vi "Create Parameters.vi"(8 "error in (no error)":errorcluster, 10 "Parameters":cluster{"Name":string, "Value":string}[](array[cluster]), 11 "XML Handler in":refnum<class "XML Handler.lvclass">) -> (0 "error out":errorcluster, 3 "XML Handler out":refnum<class "XML Handler.lvclass">)   [LabVIEW 2020, in "XML Handler.lvclass"]
uses:
  XML Handler.lvclass
  XML Handler.lvclass/XML Handler.ctl
  <vilib>/xml/Close Reference(Node).vi
  <resource>/objmgr/DOMUserDefRef.rc
  <vilib>/xml/NI_XML.lvlib
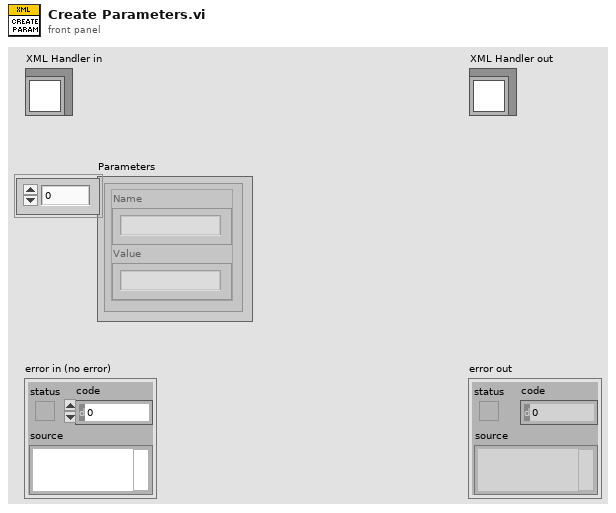
[diagram p1: front panel]
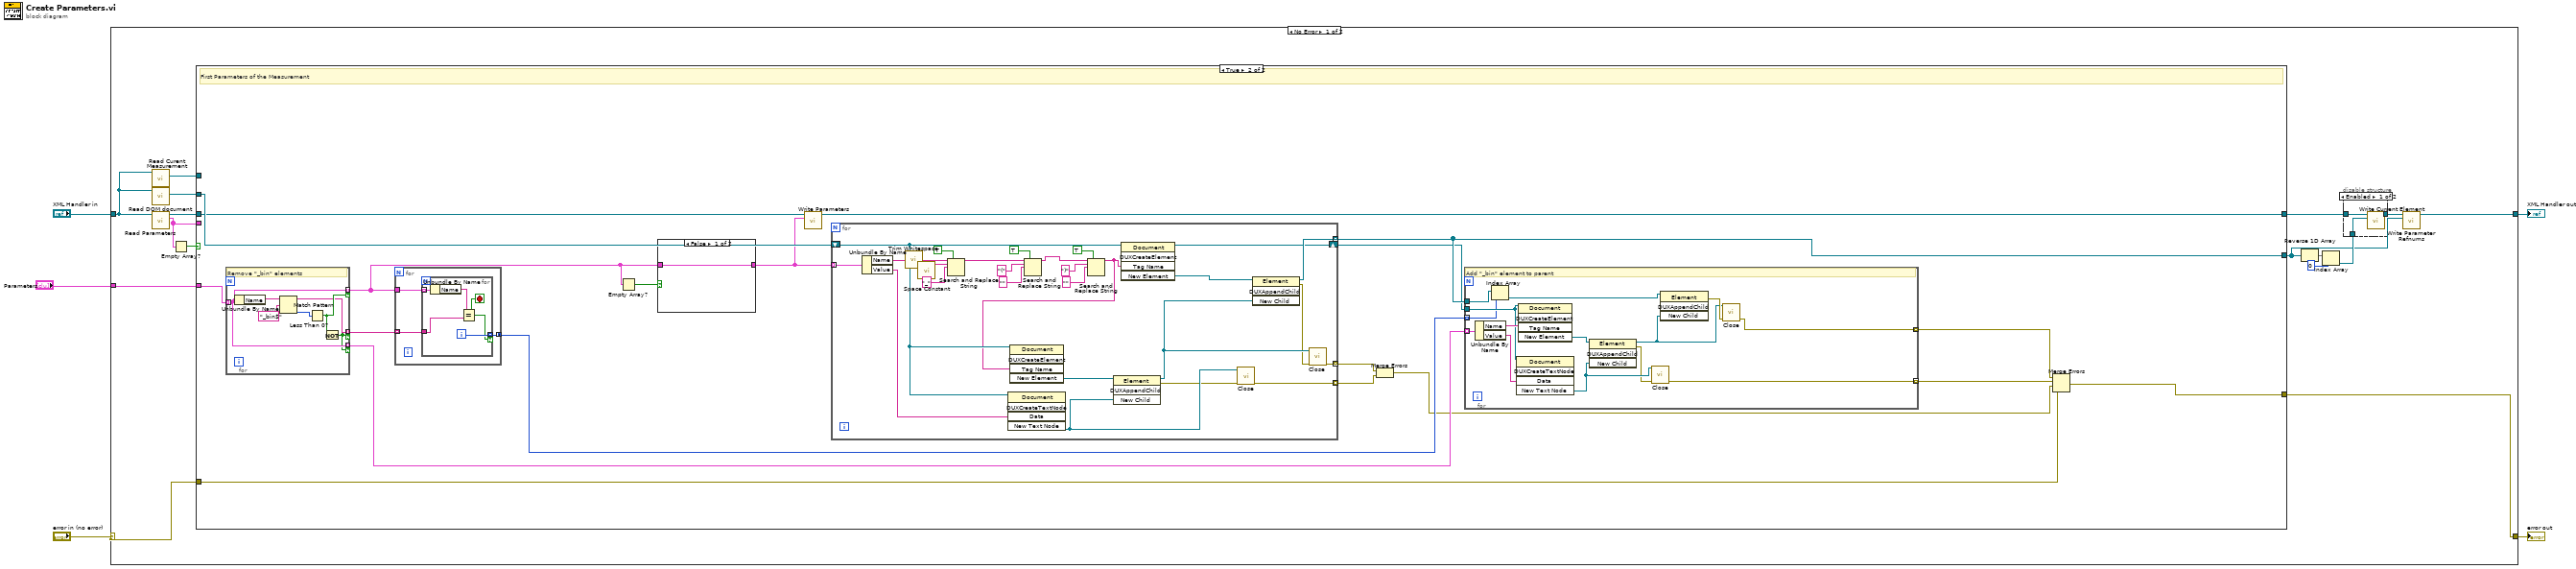
[diagram p0: block diagram]
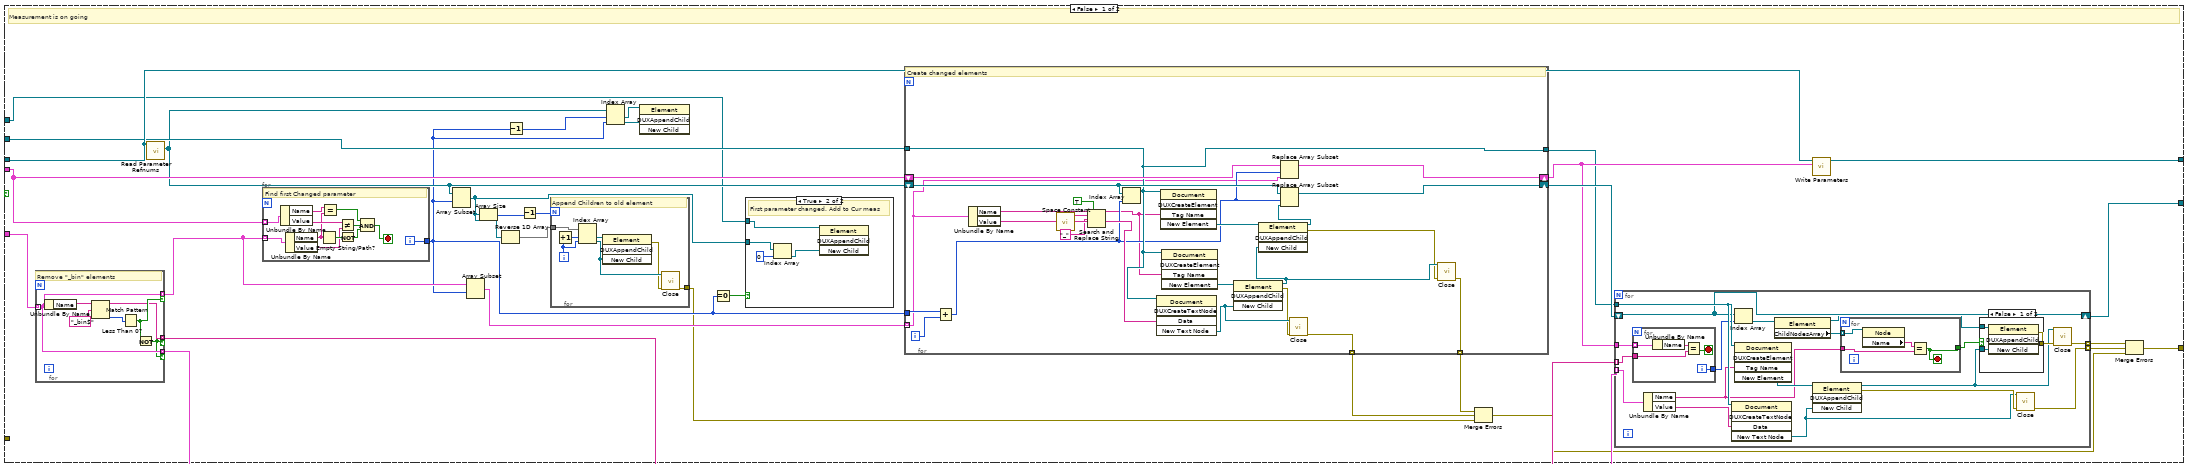
[diagram p3: hidden frame]
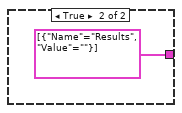
[diagram p6: hidden frame]
diagram:
  n1 = case shown="No Error" "error in (no error)" {
    selector: "error in (no error)" -> [w7 w220]
    tunnel: [w6 w220] -> w4
    tunnel: [w11 w219] -> w2
    tunnel: "XML Handler in" -> [w21 w219]
    tunnel: "Parameters" -> [w20 _]
    frame No Error {
      n2 = call "Read Curent Measurement.vi"("XML Handler in"=w21) -> ("Curent Measurement"=w13:refnum<k20>)  [unwired: 9 in, 1 out]
      n3 = call "Read DOM document.vi"("XML Handler in"=w21) -> ("DOM document"=w15:refnum<k20>)  [unwired: 9 in, 1 out]
      n4 = call "Read Parameters.vi"("XML Handler in"=w21) -> ("Parameters"=w14:cluster{"Name":string, "Value":string}[], "XML Handler out"=w16:refnum<class "XML Handler.lvclass">)  [unwired: 9 in]
      n5 = Empty Array?(array=w14) -> (empty?=w17:bool)
      n6 = case shown="True" w17 {
        tunnel: w16 -> [w55 w159]
        tunnel: w20 -> [w54 w157]
        tunnel: w15 -> [w52 w160]
        tunnel: [w50 w153] -> w10
        tunnel: [w56 w158] -> w18
        tunnel: w14 -> [w53 _]
        tunnel: w13 -> [w34 _]
        tunnel: w7 -> [_ w143]
        tunnel: [w27 w142] -> w6
        frame False {
          # "Measurement is on going"
          n7 = for {
            tunnel: w54 -> [w101] mode=indexing
            tunnel: [w101] -> w45 mode=indexing if=w102
            tunnel: [w101] -> w47 mode=indexing if=w99
            tunnel: [w100] -> w48 mode=indexing if=w99
            # "Remove \"_bin\" elements"
            n8 = Unbundle By Name(w101) -> ("Name"=w105:string)
            n9 = Match Pattern(string=w105, regular expression="_bin$") -> (before substring=w100:string, offset past match=w103:i32)  [unwired: 1 in, 2 out]
            n10 = Less Than 0?(x=w103) -> (x < 0?=w102:bool)
            n11 = Not(x=w102) -> (.not. x?=w99:bool)
          }
          n12 = call "Read Parameter Refnums.vi"("XML Handler in"=w55) -> ("Parameter Refnums"=w41:refnum<k20>[])  [unwired: 9 in, 1 out]
          n13 = for {
            tunnel: w53 -> [w137] mode=indexing
            tunnel: w45 -> [w132] mode=indexing
            tunnel: [w138] -> w37
            i -> [w138]
            stop <- w130 stop-if-true
            # "Find first Changed parameter"
            n14 = Unbundle By Name(w137) -> ("Name"=w134:string, "Value"=w135:string)
            n15 = Unbundle By Name(w132) -> ("Name"=w131:string, "Value"=w136:string)
            n16 = Empty String/Path?(string/path=w131) -> (empty?=w141:bool)
            n17 = Equal?(x=w134, y=w131) -> (x = y?=w133:bool)
            n18 = Not Equal?(x=w135, y=w136) -> (x != y?=w139:bool)
            n19 = Not(x=w141) -> (.not. x?=w140:bool)
            n20 = Compound Arithmetic op=AND(w133, w139, w140) -> (w130:bool)
          }
          n21 = Array Subset(array=w41, index=w37) -> (w35:refnum<k20>[])  [unwired: 1 in]
          n22 = Array Subset(array=w45, index=w37) -> (w42:cluster{"Name":string, "Value":string}[])  [unwired: 1 in]
          n23 = Array Size(array=w35) -> (size(s)=w44:i32)
          n24 = Reverse 1D Array(array=w35) -> (reversed array=w43:refnum<k20>[])
          n25 = Decrement(x=w37) -> (x-1=w40:i32)
          n26 = Decrement(x=w44) -> (x-1=w26:i32)
          n27 = for {
            N: w26 -> [_]
            tunnel: w43 -> [w67]
            tunnel: [w61] -> w31
            i -> [w65]
            # "Append Children to old element"
            n28 = Increment(x=w65) -> (x+1=w66:i32)
            n29 = Index Array(array=w67, index #1=w66, index #2=w65) -> (element #1=w64:refnum<k20>, element #2=w63:refnum<k20>)
            n30 = invoke class="Element" method="DUXAppendChild"(reference=w64, "New Child"=w63) -> (error out=w62:errorcluster)  [unwired: 2 in, 3 out]
            n31 = call-poly <vilib>:"Close.vi"("error in (no error)"=w62, "node"=w63) -> ("error out"=w61:errorcluster)  [unwired: 7 in]
          }
          n32 = Index Array(array=w41, index #1=w40, index #2=w37) -> (element #1=w39:refnum<k20>, element #2=w38:refnum<k20>)
          n33 = invoke class="Element" method="DUXAppendChild"(reference=w39, "New Child"=w38) -> ()  [unwired: 2 in, 4 out]
          n34 = Equal To 0?(x=w37) -> (x = 0?=w36:bool)
          n35 = case shown="True" w36 {
            tunnel: w35 -> [_ w59]
            tunnel: w34 -> [_ w60]
            frame False {
            }
            frame True {
              # "First parameter changed. Add to Cur meas"
              n36 = Index Array(array=w59, index=0) -> (element=w57:refnum<k20>)
              n37 = invoke class="Element" method="DUXAppendChild"(reference=w60, "New Child"=w57) -> ()  [unwired: 2 in, 4 out]
            }
          }
          n38 = for {
            tunnel: w52 -> [w125]
            shift-right: [w128] -> w51
            shift-left: w41 -> [w129]
            shift-right: [w126] -> w49
            shift-left: w53 -> [w127]
            tunnel: [w125] -> w46
            tunnel: w42 -> [w113] mode=indexing
            tunnel: w37 -> [w116]
            tunnel: [w112] -> w33 mode=indexing
            tunnel: [w111] -> w32 mode=indexing
            i -> [w115]
            # "Create changed elements"
            n39 = Add(x=w116, y=w115) -> (x+y=w114:i32)
            n40 = Unbundle By Name(w113) -> ("Name"=w107:string, "Value"=w124:string)
            n41 = call <vilib>:"Space Constant.vi"() -> ("String"=w109:string)
            n42 = Search and Replace String(replace all?=TRUE ("replace all? (F)"), input string=w107, search string=w109, replace string="_") -> (result string=w106:string)  [unwired: 4 in, 3 out]
            n43 = Index Array(array=w129, index=w114) -> ()  [unwired: 1 out]
            n44 = invoke class="Document" method="DUXCreateTextNode"(reference=w125, "Data"=w124) -> ("New Text Node"=w120:refnum<k20>)  [unwired: 3 in, 4 out]
            n45 = invoke class="Document" method="DUXCreateElement"(reference=w125, "Tag Name"=w106) -> ("New Element"=w123:refnum<k20>)  [unwired: 3 in, 4 out]
            n46 = invoke class="Document" method="DUXCreateElement"(reference=w125, "Tag Name"=w106) -> ("New Element"=w121:refnum<k20>)  [unwired: 3 in, 4 out]
            n47 = invoke class="Element" method="DUXAppendChild"(reference=w121, "New Child"=w120) -> (reference out=w118:refnum<k20>, error out=w119:errorcluster)  [unwired: 2 in, 2 out]
            n48 = invoke class="Element" method="DUXAppendChild"(reference=w123, "New Child"=w118) -> (reference out=w122:refnum<k20>, error out=w117:errorcluster)  [unwired: 2 in, 2 out]
            n49 = Replace Array Subset(array=w127, new element=w113, index=w114) -> (w126:cluster{"Name":string, "Value":string}[])
            n50 = Replace Array Subset(array=w129, new element=w122, index=w114) -> (w128:refnum<k20>[])
            n51 = call-poly <vilib>:"Close.vi"("error in (no error)"=w119, "node"=w120) -> ("error out"=w111:errorcluster)  [unwired: 7 in]
            n52 = call-poly <vilib>:"Close.vi"("error in (no error)"=w117, "node"=w118) -> ("error out"=w112:errorcluster)  [unwired: 7 in]
          }
          n53 = Merge Errors(w33, w32, w31) -> (w30:errorcluster)
          n54 = for {
            tunnel: w49 -> [w86]
            tunnel: w47 -> [w85] mode=indexing
            shift-right: [w78] -> w50
            shift-left: w51 -> [w78]
            tunnel: w46 -> [w84]
            tunnel: w48 -> [w75] mode=indexing
            tunnel: [w69] -> w29 mode=indexing
            tunnel: [w68] -> w28 mode=indexing
            n55 = for {
              tunnel: w75 -> [w96]
              tunnel: w86 -> [w98] mode=indexing
              tunnel: [w94] -> w79
              i -> [w94]
              stop <- w95 stop-if-true
              n56 = Unbundle By Name(w98) -> ("Name"=w97:string)
              n57 = Equal?(x=w97, y=w96) -> (x = y?=w95:bool)
            }
            n58 = Unbundle By Name(w85) -> ("Name"=w72:string, "Value"=w83:string)
            n59 = invoke class="Document" method="DUXCreateTextNode"(reference=w84, "Data"=w83) -> ("New Text Node"=w80:refnum<k20>)  [unwired: 3 in, 4 out]
            n60 = Index Array(array=w78, index=w79) -> (element=w74:refnum<k20>)
            n61 = invoke class="Document" method="DUXCreateElement"(reference=w84, "Tag Name"=w72) -> ("New Element"=w82:refnum<k20>)  [unwired: 3 in, 4 out]
            n62 = property class="Element"(reference=w74) -> (reference out=w71:refnum<k20>, "ChildNodesArray"=w73:refnum<k20>[])  [unwired: 1 in, 1 out]
            n63 = invoke class="Element" method="DUXAppendChild"(reference=w82, "New Child"=w80) -> (reference out=w76:refnum<k20>, error out=w81:errorcluster)  [unwired: 2 in, 2 out]
            n64 = for {
              tunnel: w73 -> [w93] mode=indexing
              tunnel: w72 -> [w91]
              tunnel: [w90] -> w70
              stop <- w90 stop-if-true
              n65 = property class="Node"(reference=w93) -> ("Name"=w92:string)  [unwired: 1 in, 2 out]
              n66 = Equal?(x=w92, y=w91) -> (x = y?=w90:bool)
            }
            n67 = case shown="False" w70 {
              tunnel: [w89 _] -> w77
              tunnel: w76 -> [w88 _]
              tunnel: w71 -> [w87 _]
              frame False {
                n68 = invoke class="Element" method="DUXAppendChild"(reference=w87, "New Child"=w88) -> (error out=w89:errorcluster)  [unwired: 2 in, 3 out]
              }
              frame True {
              }
            }
            n69 = call-poly <vilib>:"Close.vi"("error in (no error)"=w81, "node"=w80) -> ("error out"=w69:errorcluster)  [unwired: 7 in]
            n70 = call-poly <vilib>:"Close.vi"("error in (no error)"=w77, "node"=w76) -> ("error out"=w68:errorcluster)  [unwired: 7 in]
          }
          n71 = call "Write Parameters.vi"("Parameters"=w49, "XML Handler in"=w55) -> ("XML Handler out"=w56:refnum<class "XML Handler.lvclass">)  [unwired: 9 in]
          n72 = Merge Errors(w28, w29, w30) -> (w27:errorcluster)
        }
        frame True {
          # "First Parameters of the Measurement"
          n73 = for {
            tunnel: w157 -> [w187] mode=indexing
            tunnel: [w187] -> w150 mode=indexing if=w188
            tunnel: [w187] -> w155 mode=indexing if=w185
            tunnel: [w186] -> w156 mode=indexing if=w185
            # "Remove \"_bin\" elements"
            n74 = Unbundle By Name(w187) -> ("Name"=w191:string)
            n75 = Match Pattern(string=w191, regular expression="_bin$") -> (before substring=w186:string, offset past match=w189:i32)  [unwired: 1 in, 2 out]
            n76 = Less Than 0?(x=w189) -> (x < 0?=w188:bool)
            n77 = Not(x=w188) -> (.not. x?=w185:bool)
          }
          n78 = for {
            tunnel: w150 -> [w178]
            tunnel: w156 -> [w179] mode=indexing
            tunnel: [w177] -> w154 mode=concatenating
            n79 = for {
              tunnel: w179 -> [w182]
              tunnel: w178 -> [w184] mode=indexing
              tunnel: [w181] -> w177 mode=indexing if=w180
              i -> [w181]
              stop <- w180 stop-if-true
              n80 = Unbundle By Name(w184) -> ("Name"=w183:string)
              n81 = Equal?(x=w183, y=w182) -> (x = y?=w180:bool)
            }
          }
          n82 = Empty Array?(array=w150) -> (empty?=w151:bool)
          n83 = case shown="False" w151 {
            tunnel: [w161 cluster{"Name":string, "Value":string}[] [{"Name"="Results", "Value"=""}]] -> w149
            tunnel: w150 -> [w161 _]
            frame False {
            }
            frame True {
            }
          }
          n84 = call "Write Parameters.vi"("Parameters"=w149, "XML Handler in"=w159) -> ("XML Handler out"=w158:refnum<class "XML Handler.lvclass">)  [unwired: 9 in]
          n85 = for {
            tunnel: w149 -> [w215] mode=indexing
            tunnel: [w217] -> w153 mode=indexing
            shift-right: [w208] -> w152
            shift-left: w160 -> [w216]
            tunnel: [w204] -> w148 mode=indexing
            tunnel: [w203] -> w147 mode=indexing
            n86 = Unbundle By Name(w215) -> ("Name"=w202:string, "Value"=w214:string)
            n87 = call <vilib>:"Trim Whitespace.vi"("string"=w202) -> ("trimmed string"=w201:string)  [unwired: 1 in]
            n88 = call <vilib>:"Space Constant.vi"() -> ("String"=w206:string)
            n89 = Search and Replace String(replace all?=TRUE ("replace all? (F)"), input string=w201, search string=w206, replace string="_") -> (result string=w193:string)  [unwired: 4 in, 3 out]
            n90 = invoke class="Document" method="DUXCreateTextNode"(reference=w216, "Data"=w214) -> ("New Text Node"=w212:refnum<k20>)  [unwired: 3 in, 4 out]
            n91 = Search and Replace String(replace all?=TRUE ("replace all? (F)"), input string=w193, search string="(", replace string="") -> (result string=w194:string)  [unwired: 4 in, 3 out]
            n92 = Search and Replace String(replace all?=TRUE ("replace all? (F)"), input string=w194, search string=")", replace string="") -> (result string=w192:string)  [unwired: 4 in, 3 out]
            n93 = invoke class="Document" method="DUXCreateElement"(reference=w216, "Tag Name"=w192) -> ("New Element"=w213:refnum<k20>)  [unwired: 3 in, 4 out]
            n94 = invoke class="Element" method="DUXAppendChild"(reference=w213, "New Child"=w212) -> (reference out=w210:refnum<k20>, error out=w211:errorcluster)  [unwired: 2 in, 2 out]
            n95 = invoke class="Document" method="DUXCreateElement"(reference=w216, "Tag Name"=w192) -> (reference out=w208:refnum<k20>, "New Element"=w218:refnum<k20>)  [unwired: 3 in, 3 out]
            n96 = call-poly <vilib>:"Close.vi"("error in (no error)"=w211, "node"=w212) -> ("error out"=w203:errorcluster)  [unwired: 7 in]
            n97 = invoke class="Element" method="DUXAppendChild"(reference=w218, "New Child"=w210) -> (reference out=w217:refnum<k20>, error out=w209:errorcluster)  [unwired: 2 in, 2 out]
            n98 = call-poly <vilib>:"Close.vi"("error in (no error)"=w209, "node"=w210) -> ("error out"=w204:errorcluster)  [unwired: 7 in]
          }
          n99 = Merge Errors(w148, w147) -> (w146:errorcluster)
          n100 = for {
            tunnel: w154 -> [w168] mode=indexing
            tunnel: w153 -> [w169]
            tunnel: w155 -> [w176] mode=indexing
            tunnel: w152 -> [w174]
            tunnel: [w164] -> w144 mode=indexing
            tunnel: [w163] -> w145 mode=indexing
            # "Add \"_bin\" element to parent"
            n101 = Unbundle By Name(w176) -> ("Name"=w175:string, "Value"=w173:string)
            n102 = Index Array(array=w169, index=w168) -> (element=w167:refnum<k20>)
            n103 = invoke class="Document" method="DUXCreateTextNode"(reference=w174, "Data"=w173) -> ("New Text Node"=w171:refnum<k20>)  [unwired: 3 in, 4 out]
            n104 = invoke class="Document" method="DUXCreateElement"(reference=w174, "Tag Name"=w175) -> ("New Element"=w172:refnum<k20>)  [unwired: 3 in, 4 out]
            n105 = invoke class="Element" method="DUXAppendChild"(reference=w172, "New Child"=w171) -> (reference out=w165:refnum<k20>, error out=w170:errorcluster)  [unwired: 2 in, 2 out]
            n106 = call-poly <vilib>:"Close.vi"("error in (no error)"=w170, "node"=w171) -> ("error out"=w163:errorcluster)  [unwired: 7 in]
            n107 = invoke class="Element" method="DUXAppendChild"(reference=w167, "New Child"=w165) -> (error out=w166:errorcluster)  [unwired: 2 in, 3 out]
            n108 = call-poly <vilib>:"Close.vi"("error in (no error)"=w166, "node"=w165) -> ("error out"=w164:errorcluster)  [unwired: 7 in]
          }
          n109 = Merge Errors(w144, w145, w146, w143) -> (w142:errorcluster)
        }
      }
      n110 = Reverse 1D Array(array=w10) -> (reversed array=w9:refnum<k20>[])
      n111 = Index Array(array=w9, index=0) -> (element=w19:refnum<k20>)
      n112 = disable-structure shown="Enabled" {
        disable-tunnel: w19 -> [w24 _]
        disable-tunnel: w18 -> [w23 w25]
        disable-tunnel: [w22 w25] -> w12
        frame Enabled {
          n113 = call "Write Current Element.vi"("Current Element"=w24, "XML Handler in"=w23) -> ("XML Handler out"=w22:refnum<class "XML Handler.lvclass">)  [unwired: 9 in]
        }
        frame Disabled {
        }
      }
      n114 = call "Write Parameter Refnums.vi"("Parameter Refnums"=w10, "XML Handler in"=w12) -> ("XML Handler out"=w11:refnum<class "XML Handler.lvclass">)  [unwired: 9 in]
    }
    frame Error {
    }
  }
  "error out" <- w4
  "XML Handler out" <- w2
